vi "Evaluate Alarms.vi"(0 "In Test":bool, 1 "Controller":T2, 2 "Alarm Config":T3, 3 "Data":dbl[](array[numeric]), 4 "Pumps Present":u32, 5 "Trip Counter":i32[](array[numeric]), 6 "Previous Times":u32[](array[numeric]), 7 "Manual CMDs":dbl[](array[numeric]), 9 "Prev ON Times":u32[](array[numeric])) -> (20 "Trip Counter OUT":i32[](array[numeric]), 21 "Previous Times OUT":u32[](array[numeric]), 22 "Alarm Tripped":bool, 24 "Prev ON Times OUT":u32[](array[numeric]), 25 "Alarm Message 1":string, 26 "Alarm Message 2":string)   [LabVIEW 2013]
uses:
  Controls/Alarm Config.ctl
  Controls/Alarm Definition.ctl
  Controls/Alarm Profile Config.ctl
  Type Defs/Controller Names.ctl
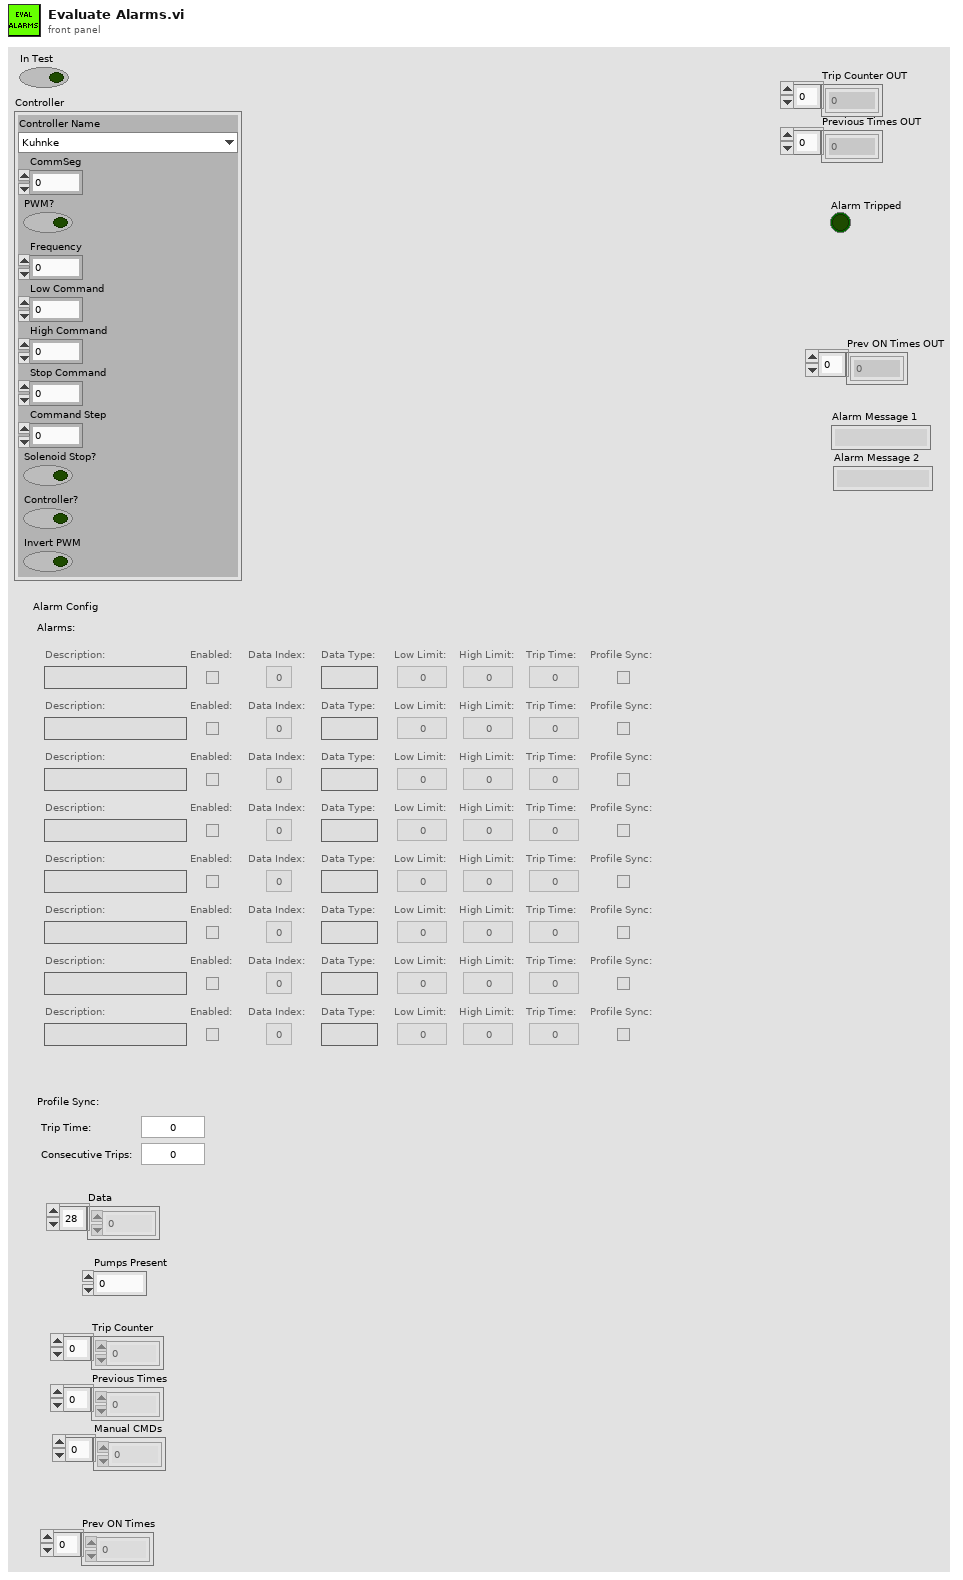
[diagram p1: front panel]
types:
  T1 = typedef "Controller Names.ctl" = enum16{"Kuhnke", "Helbako BLDC", "Conti", "Hella BLDC OL PWM", "Hella BLDC Turbine OL PWM", "Hella BLDC Pressure", "Helbako (old)", "TI PWM", "PSA", "Hella Gas", "Hella Diesel", "8 Comm", "10 Comm", "8 Comm Hella", "10 Comm Hella", "8 Comm Omron", "10 Comm Omron", "8 Comm Nissan", "10 Comm Nissan"}
  T2 = cluster{"Controller Name":T1, "CommSeg":i32, "PWM?":bool, "Frequency":i32, "Low Command":dbl, "High Command":dbl, "Stop Command":dbl, "Command Step":dbl, "Solenoid Stop?":bool, "Controller?":bool, "Invert PWM":bool}
  T3 = typedef "Alarm Config.ctl" = cluster{"Alarms:":T4[], "Profile Sync:":T5}
  T4 = typedef "Alarm Definition.ctl" = cluster{"Description:":string, "Enabled:":bool, "Data Index:":i32, "Data Type:":string, "Low Limit:":dbl, "High Limit:":dbl, "Trip Time:":u32, "Profile Sync:":bool}
  T5 = typedef "Alarm Profile Config.ctl" = cluster{"Trip Time:":u32, "Consecutive Trips:":i32}
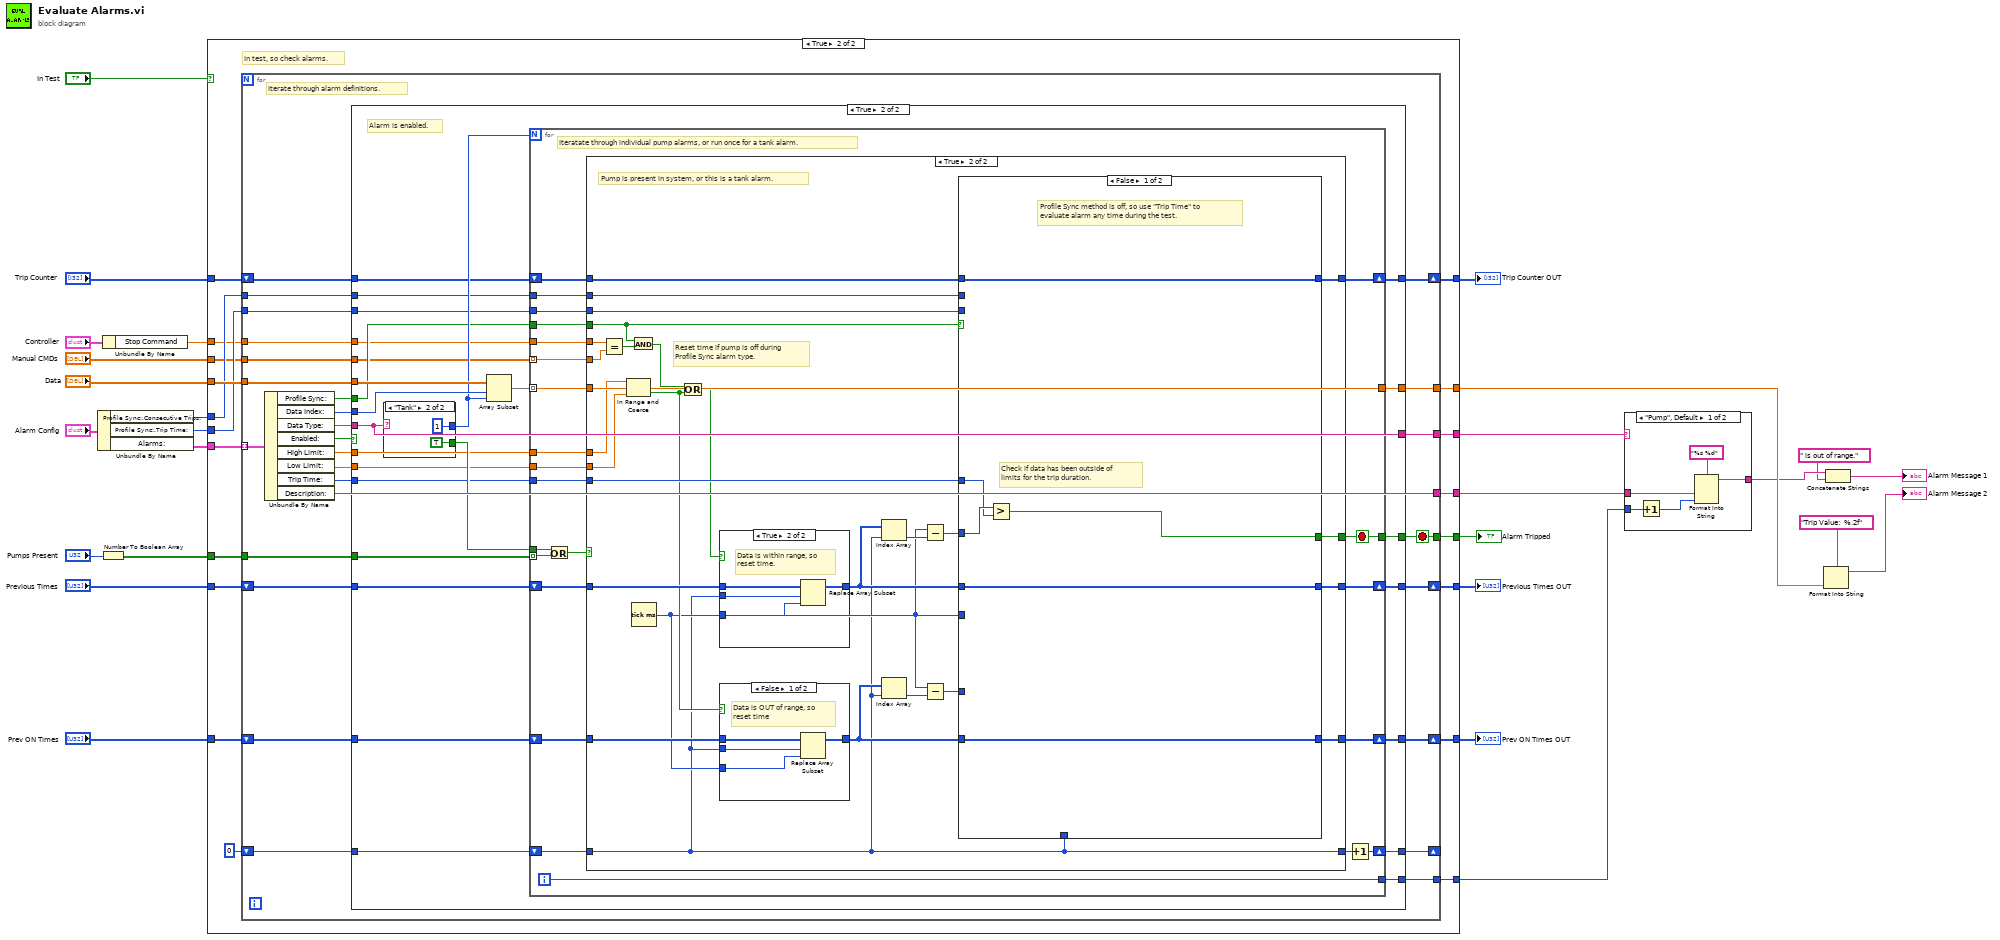
[diagram p0: block diagram]
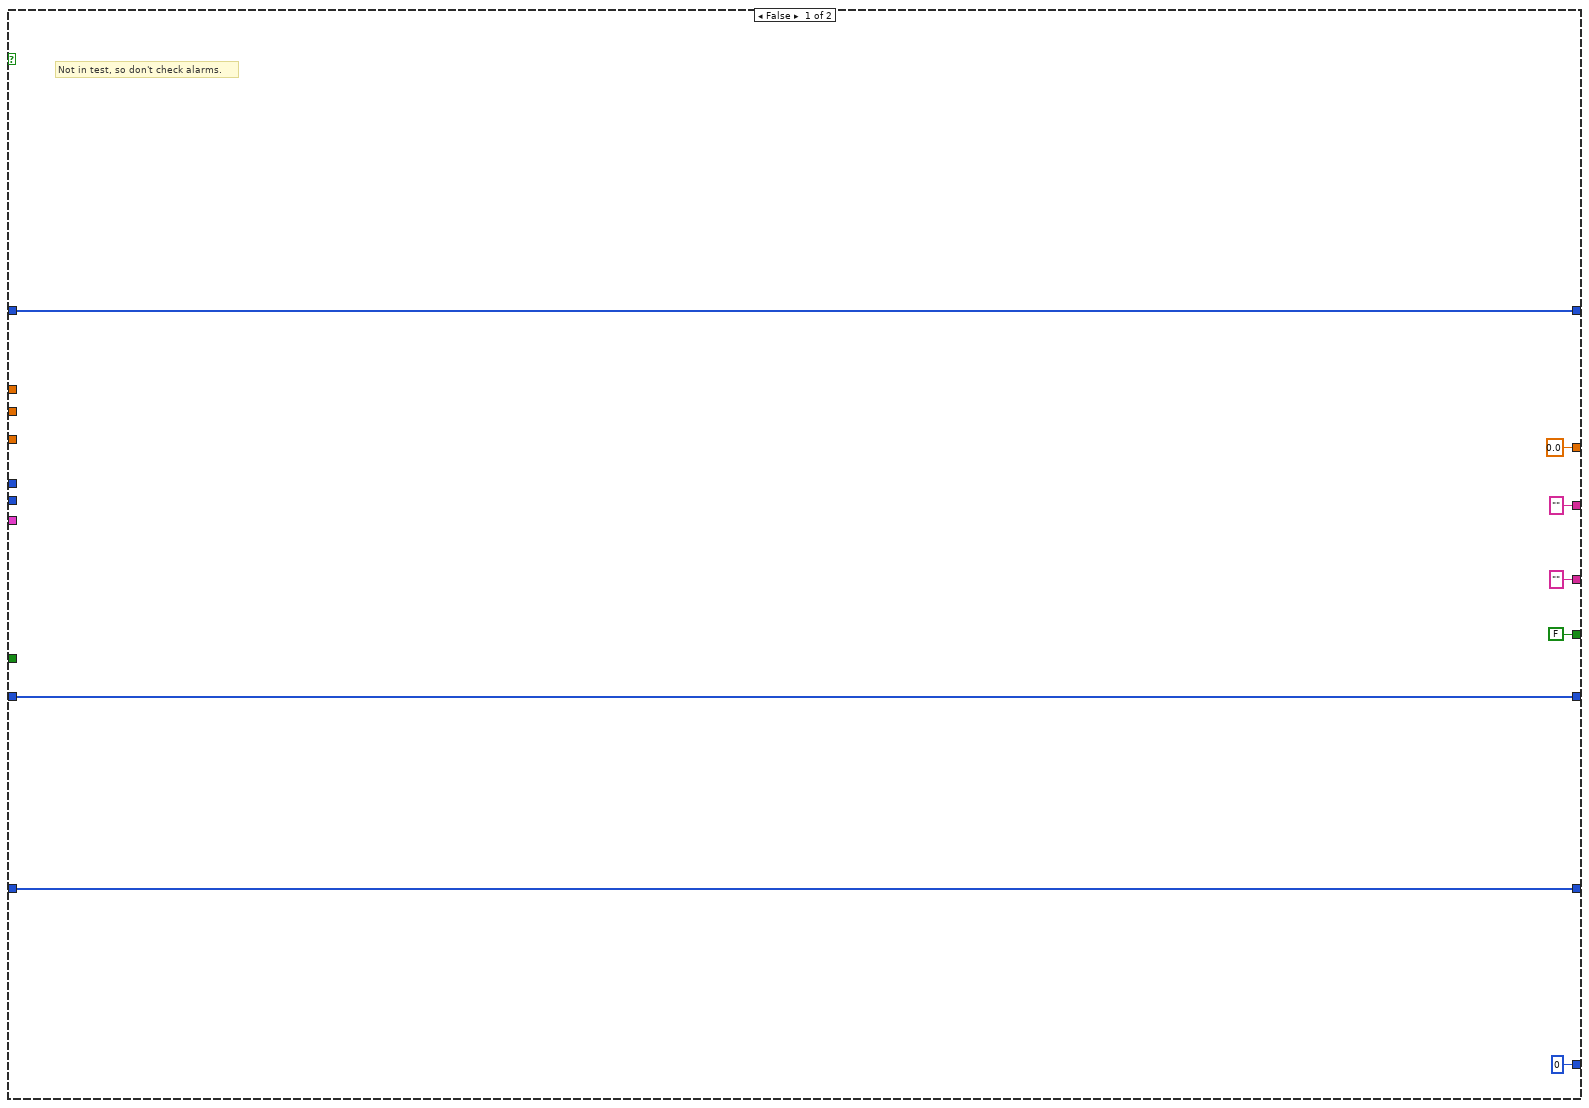
[diagram p3: hidden frame]
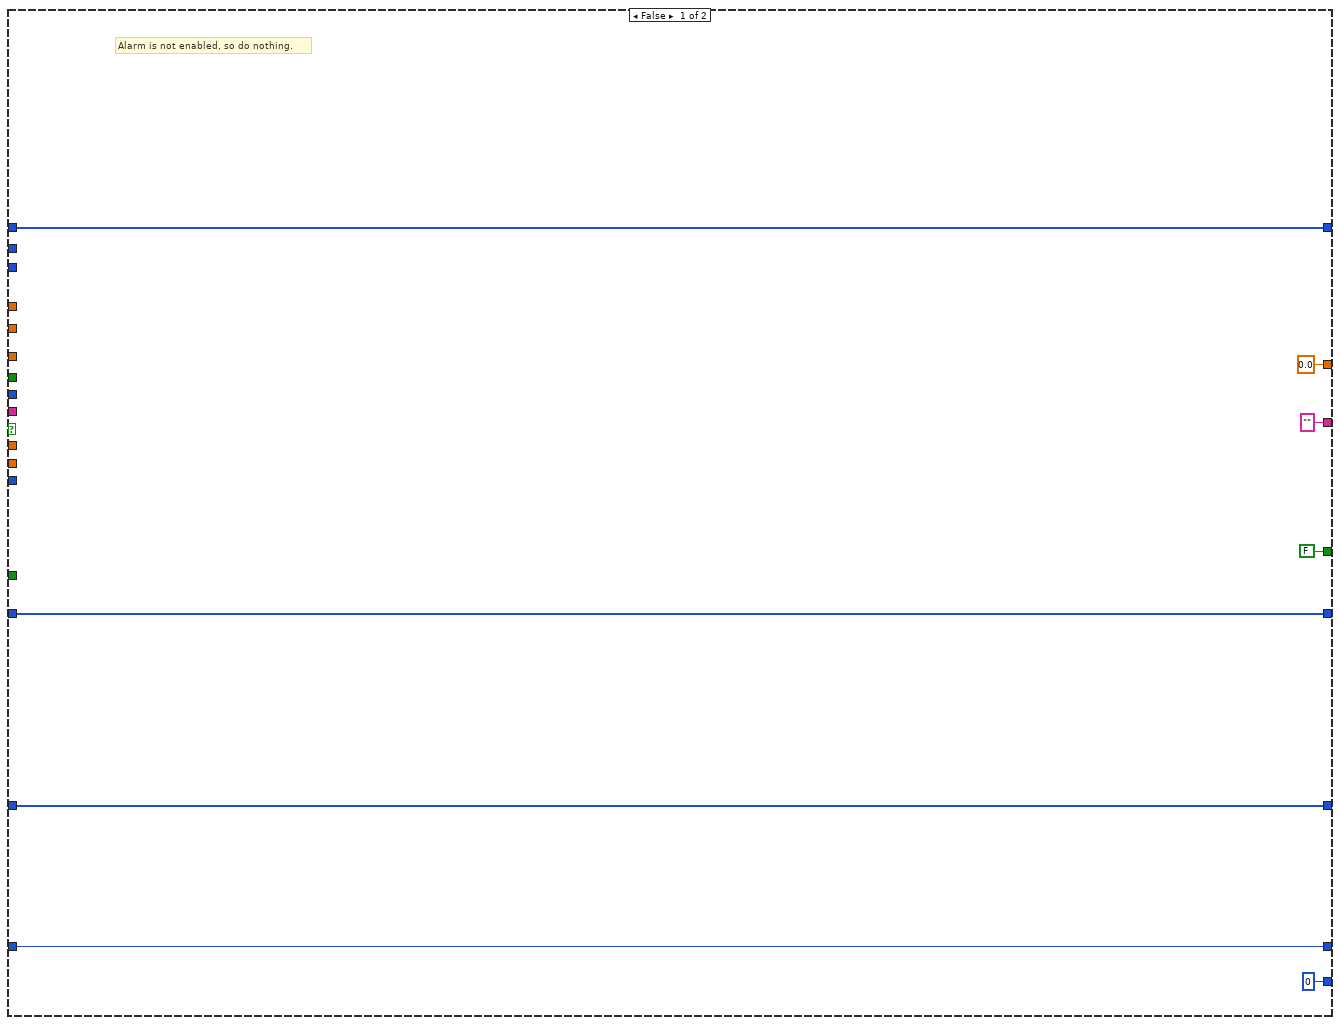
[diagram p4: hidden frame]
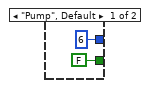
[diagram p5: hidden frame]
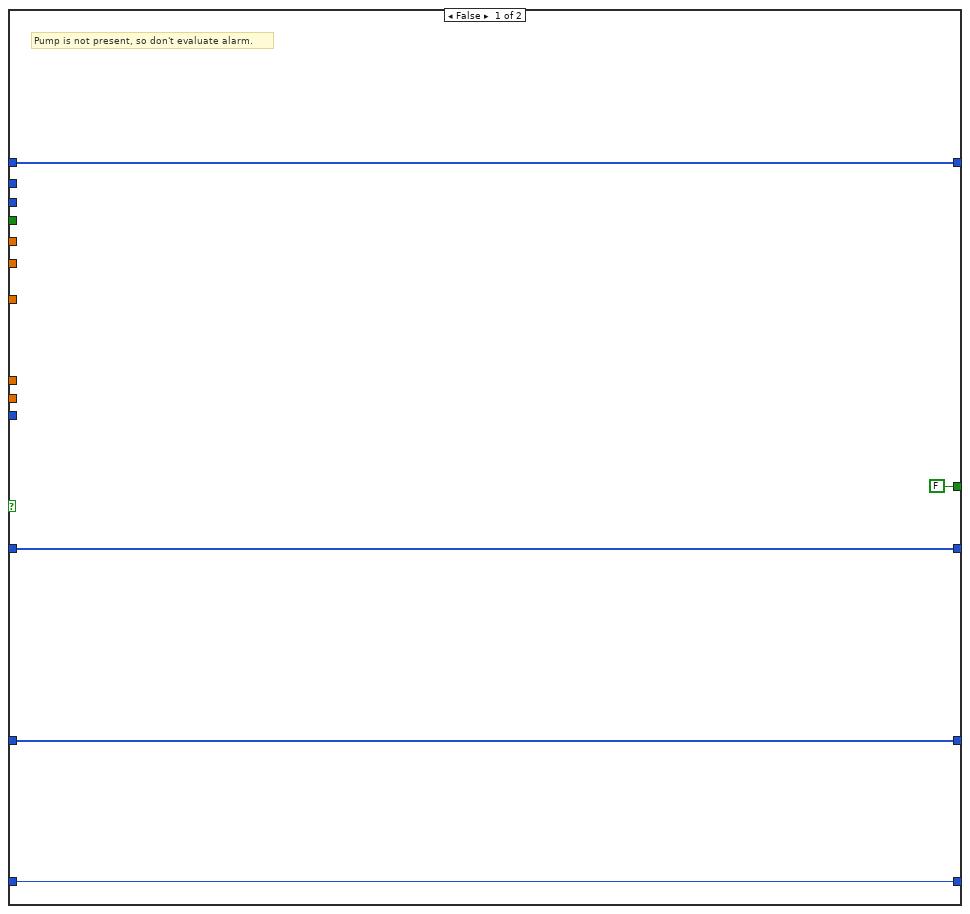
[diagram p6: hidden frame]
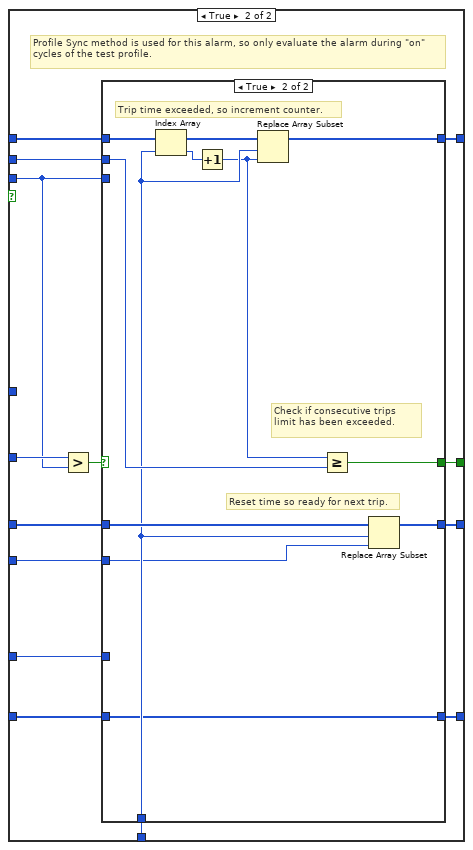
[diagram p9: hidden frame]
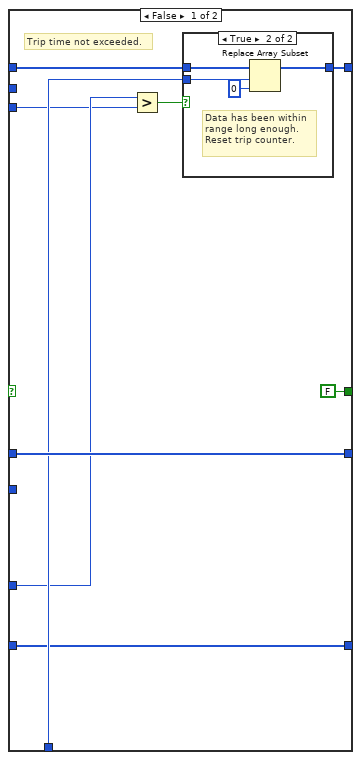
[diagram p10: hidden frame]
diagram:
  n1 = Unbundle By Name("Alarm Config") -> ("Profile Sync:.Consecutive Trips:"=w19:i32, "Profile Sync:.Trip Time:"=w18:u32, "Alarms:"=w24:T4[])
  n2 = Number To Boolean Array(number="Pumps Present") -> (Boolean array=w21:bool[])
  n3 = Unbundle By Name("Controller") -> ("Stop Command"=w17:dbl)
  n4 = case shown="True" "In Test" {
    tunnel: w24 -> [_ w54]
    tunnel: "Data" -> [_ w53]
    tunnel: w21 -> [_ w52]
    tunnel: "Previous Times" -> [w34 w51]
    tunnel: "Trip Counter" -> [w35 w49]
    tunnel: w19 -> [_ w48]
    tunnel: w18 -> [_ w47]
    tunnel: w17 -> [_ w46]
    tunnel: "Manual CMDs" -> [_ w45]
    tunnel: [w35 w44] -> w14
    tunnel: [w34 w43] -> w13
    tunnel: [FALSE w42] -> w12
    tunnel: ["" ("Description:") w41] -> w10
    tunnel: [0 w40] -> w9
    tunnel: ["" ("Data Type:") w39] -> w11
    tunnel: [0.0 w38] -> w5
    tunnel: "Prev ON Times" -> [w28 w37]
    tunnel: [w28 w36] -> w7
    frame False {
      # "Not in test, so don't check alarms."
    }
    frame True {
      # "In test, so check alarms."
      n5 = for {
        tunnel: w54 -> [w81] mode=indexing
        tunnel: w53 -> [w79]
        tunnel: w52 -> [w76]
        shift-right: [w71] -> w43
        shift-left: w51 -> [w72]
        shift-right: [w68] -> _
        shift-left: 0 ("index") -> [w69]
        shift-right: [w66] -> w44
        shift-left: w49 -> [w67]
        tunnel: w48 -> [w65]
        tunnel: w47 -> [w64]
        tunnel: w46 -> [w63]
        tunnel: w45 -> [w62]
        tunnel: [w61] -> w42
        tunnel: [w60] -> w41
        tunnel: [w59] -> w40
        tunnel: [w58] -> w39
        tunnel: [w57] -> w38
        shift-right: [w55] -> w36
        shift-left: w37 -> [w56]
        stop <- w61 stop-if-true
        # "Iterate through alarm definitions."
        n6 = Unbundle By Name(w81) -> ("Profile Sync:"=w70:bool, "Data Index:"=w78:i32, "Data Type:"=w77:string, "Enabled:"=w80:bool, "High Limit:"=w75:dbl, "Low Limit:"=w74:dbl, "Trip Time:"=w73:u32, "Description:"=w60:string)
        n7 = case shown="True" w80 {
          tunnel: w79 -> [_ w115]
          tunnel: w78 -> [_ w114]
          tunnel: w77 -> [_ w93]
          tunnel: w76 -> [_ w111]
          tunnel: w75 -> [_ w110]
          tunnel: w74 -> [_ w109]
          tunnel: w73 -> [_ w108]
          tunnel: w72 -> [w87 w106]
          tunnel: [w87 w105] -> w71
          tunnel: w70 -> [_ w104]
          tunnel: w69 -> [w86 w103]
          tunnel: [w86 w102] -> w68
          tunnel: [FALSE w101] -> w61
          tunnel: w67 -> [w89 w100]
          tunnel: [w89 w99] -> w66
          tunnel: w65 -> [_ w98]
          tunnel: w64 -> [_ w97]
          tunnel: w63 -> [_ w96]
          tunnel: w62 -> [_ w95]
          tunnel: [0 w94] -> w59
          tunnel: ["" ("Data Type:") w93] -> w58
          tunnel: [0.0 w92] -> w57
          tunnel: w56 -> [w82 w91]
          tunnel: [w82 w90] -> w55
          frame False {
            # "Alarm is not enabled, so do nothing."
          }
          frame True {
            # "Alarm is enabled."
            n8 = case shown="\"Tank\"" w93 {
              tunnel: [6 ("length") 1 ("length")] -> w113
              tunnel: [FALSE TRUE] -> w112
              frame "Pump", Default {
              }
              frame "Tank" {
              }
            }
            n9 = Array Subset(array=w115, index=w114, length=w113) -> (w107:dbl[])
            n10 = for {
              N: w113 -> [_]
              tunnel: w112 -> [w142]
              tunnel: w111 -> [w141] mode=indexing
              tunnel: w110 -> [w139]
              tunnel: w109 -> [w138]
              tunnel: w108 -> [w137]
              tunnel: w107 -> [w123] mode=indexing
              shift-right: [w135] -> w105
              shift-left: w106 -> [w136]
              tunnel: w104 -> [w134]
              shift-right: [w124] -> w102
              shift-left: w103 -> [w133]
              tunnel: [w132] -> w101
              shift-right: [w130] -> w99
              shift-left: w100 -> [w131]
              tunnel: w98 -> [w129]
              tunnel: w97 -> [w128]
              tunnel: w96 -> [w127]
              tunnel: w95 -> [w126] mode=indexing
              tunnel: [w120] -> w94
              tunnel: [w123] -> w92
              shift-right: [w121] -> w90
              shift-left: w91 -> [w122]
              i -> [w120]
              stop <- w132 stop-if-true
              # "Iteratate through individual pump alarms, or run once for a tank alarm."
              n11 = Or(x=w142, y=w141) -> (x .or. y?=w140:bool)
              n12 = case shown="True" w140 {
                tunnel: w139 -> [_ w175]
                tunnel: w138 -> [_ w174]
                tunnel: w137 -> [_ w170]
                tunnel: w123 -> [_ w149]
                tunnel: w136 -> [w145 w173]
                tunnel: [w145 w158] -> w135
                tunnel: w134 -> [_ w162]
                tunnel: w133 -> [w144 w148]
                tunnel: [w144 w148] -> w125
                tunnel: [FALSE w171] -> w132
                tunnel: w131 -> [w147 w169]
                tunnel: [w147 w168] -> w130
                tunnel: w129 -> [_ w167]
                tunnel: w128 -> [_ w166]
                tunnel: w127 -> [_ w165]
                tunnel: w126 -> [_ w164]
                tunnel: w122 -> [w143 w156]
                tunnel: [w143 w153] -> w121
                frame False {
                  # "Pump is not present, so don't evaluate alarm."
                }
                frame True {
                  # "Reset time if pump is off during\nProfile Sync alarm type."
                  # "Pump is present in system, or this is a tank alarm."
                  n13 = Equal?(x=w165, y=w164) -> (x = y?=w163:bool)
                  n14 = In Range and Coerce(upper limit=w175, x=w149, lower limit=w174) -> (In Range?=w157:bool)  [unwired: 1 out]
                  n15 = And(x=w162, y=w163) -> (x .and. y?=w161:bool)
                  n16 = Tick Count (ms)() -> (millisecond timer value=w154:u32)
                  n17 = Or(x=w161, y=w157) -> (x .or. y?=w160:bool)
                  n18 = case shown="True" w160 {
                    tunnel: w173 -> [w181 w185]
                    tunnel: [w181 w184] -> w159
                    tunnel: w148 -> [_ w183]
                    tunnel: w154 -> [_ w182]
                    frame False {
                      # "Data is out of range, so\nmaintain previous time."
                    }
                    frame True {
                      # "Data is within range, so\nreset time."
                      n19 = Replace Array Subset(array=w185, new element=w182, index=w183) -> (w184:u32[])
                    }
                  }
                  n20 = case shown="False" w157 {
                    tunnel: w156 -> [w179 w180]
                    tunnel: [w178 w180] -> w152
                    tunnel: w148 -> [w177 _]
                    tunnel: w154 -> [w176 _]
                    frame False {
                      # "Data is OUT of range, so\nreset time"
                      n21 = Replace Array Subset(array=w179, new element=w176, index=w177) -> (w178:u32[])
                    }
                    frame True {
                      # "Data is WITHIN range, so\nmaintain previous time."
                    }
                  }
                  n22 = Index Array(array=w159, index=w148) -> (element=w172:u32)
                  n23 = Index Array(array=w152, index=w148) -> (element=w155:u32)
                  n24 = Subtract(x=w154, y=w172) -> (x-y=w151:u32)
                  n25 = Subtract(x=w154, y=w155) -> (x-y=w150:u32)
                  n26 = case shown="False" w162 {
                    tunnel: [w189 w199] -> w171
                    tunnel: w151 -> [w191 w205]
                    tunnel: w170 -> [w190 _]
                    tunnel: w169 -> [w188 w204]
                    tunnel: [w188 w203] -> w168
                    tunnel: w167 -> [_ w200]
                    tunnel: w166 -> [_ w192]
                    tunnel: w148 -> [_ w201]
                    tunnel: w159 -> [w187 w198]
                    tunnel: [w187 w197] -> w158
                    tunnel: w154 -> [_ w196]
                    tunnel: w152 -> [w186 w195]
                    tunnel: [w186 w194] -> w153
                    tunnel: w150 -> [_ w193]
                    frame False {
                      # "Check if data has been outside of\nlimits for the trip duration."
                      # "Profile Sync method is off, so use \"Trip Time\" to\nevaluate alarm any time during the test."
                      n27 = Greater?(x=w191, y=w190) -> (0:w189:bool)
                    }
                    frame True {
                      # "Profile Sync method is used for this alarm, so only evaluate the alarm during \"on\" cycles of the test profile."
                      n28 = Greater?(x=w205, y=w192) -> (0:w202:bool)
                      n29 = case shown="True" w202 {
                        tunnel: [w211 w230] -> w203
                        tunnel: w204 -> [w212 w229]
                        tunnel: w201 -> [w210 w223]
                        tunnel: w200 -> [_ w227]
                        tunnel: [FALSE w226] -> w199
                        tunnel: w198 -> [w213 w225]
                        tunnel: [w213 w224] -> w197
                        tunnel: w196 -> [_ w222]
                        tunnel: [w206 w221] -> w194
                        tunnel: w195 -> [w206 w221]
                        tunnel: w193 -> [w209 _]
                        tunnel: w192 -> [w208 _]
                        frame False {
                          # "Trip time not exceeded."
                          n30 = Greater?(x=w209, y=w208) -> (0:w207:bool)
                          n31 = case shown="True" w207 {
                            tunnel: w212 -> [w215 w219]
                            tunnel: [w215 w218] -> w211
                            tunnel: w210 -> [_ w217]
                            frame False {
                              # "Data has NOT come\ncome back into range\nlong enough.\nMaintain counters."
                            }
                            frame True {
                              # "Data has been within\nrange long enough. \nReset trip counter."
                              n32 = Replace Array Subset(array=w219, new element=0 ("new element/subarray"), index=w217) -> (w218:i32[])
                            }
                          }
                        }
                        frame True {
                          # "Reset time so ready for next trip."
                          # "Check if consecutive trips limit has been exceeded."
                          # "Trip time exceeded, so increment counter."
                          n33 = Index Array(array=w229, index=w223) -> (element=w228:i32)
                          n34 = Increment(x=w228) -> (x+1=w220:i32)
                          n35 = Replace Array Subset(array=w229, new element=w220, index=w223) -> (w230:i32[])
                          n36 = Greater Or Equal?(x=w220, y=w227) -> (x >= y?=w226:bool)
                          n37 = Replace Array Subset(array=w225, new element=w222, index=w223) -> (w224:u32[])
                        }
                      }
                    }
                  }
                }
              }
              n38 = Increment(x=w125) -> (x+1=w124:i32)
            }
          }
        }
      }
    }
  }
  "Trip Counter OUT" <- w14
  "Previous Times OUT" <- w13
  "Alarm Tripped" <- w12
  "Prev ON Times OUT" <- w7
  n39 = case shown="\"Pump\", Default" w11 {
    tunnel: w10 -> [w233 w236]
    tunnel: w9 -> [w232 _]
    tunnel: [w234 w236] -> w2
    frame "Pump", Default {
      n40 = Increment(x=w232) -> (x+1=w231:i32)
      n41 = Format Into String(format string="%s %d", w233, w231) -> (resulting string=w234:string)  [unwired: 2 in, 1 out]
    }
    frame "Tank" {
    }
  }
  n42 = Format Into String(format string="Trip Value:  %.2f", w5) -> (resulting string=→"Alarm Message 2":string)  [unwired: 2 in, 1 out]
  n43 = Concatenate Strings(w2, " is out of range." ("format string")) -> (→"Alarm Message 1":string)
